vi "Configure CAN Trigger.vi"(0 "VISA resource name":refnum<visa-resource-name>, 1 "Trigger Condition (0: Start of Frame (SOF))":i32(ring) items=["Start of Frame (SOF)", "Data", "Error", "ID Data", "ID Remote", "All Errors", "Overload", "ACK Error", "Message", "MSignal"], 5 "CAN Channel (1: Channel 1)":i32(ring)=1 items=["Channel 1"=1, "Channel 2"=2, "Channel 3"=3, "Channel 4"=4], 7 "Identifier Type (0: Standard)":i32(ring) items=["Standard", "Extended"], 9 "Data Pattern Resource":string="XXXXXXXXXXXXXXXXXXXXXXXXXXXXXXXXXXXXXXXXXXXXXXXXXXXXXXXXXXXXXXXX", 11 "error in (no error)":errorcluster, 12 "Data Pattern Length (8)":i32=8, 13 "Data Pattern ID (XXXXXXXXXXX)":string="XXXXXXXXXXX") -> (4 "VISA resource name out":refnum<visa-resource-name>, 15 "error out":errorcluster)   [LabVIEW 2013, in "Agilent 90000 Series.lvlib"]
doc: "Configures triger values for serial bus.\n\n<b>Notes:</b>\n1. You must set the proper :SBUS<N>:MODE, :SBUS<N>:CAN:TRIGger, and :SBUS<N>:CAN:TRIGger:PATTern:ID:MODE before setting any other trigger values. \n2. This VI is new in firmware version 4.60."
uses:
  Agilent 90000 Series.lvlib
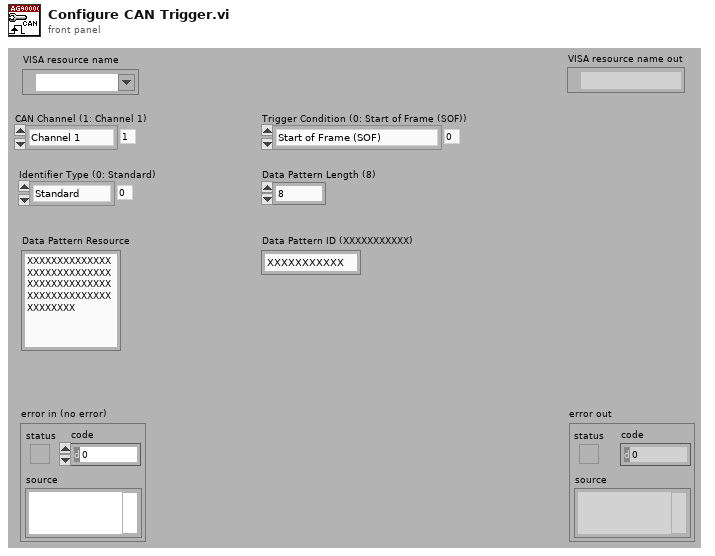
[diagram p1: front panel]
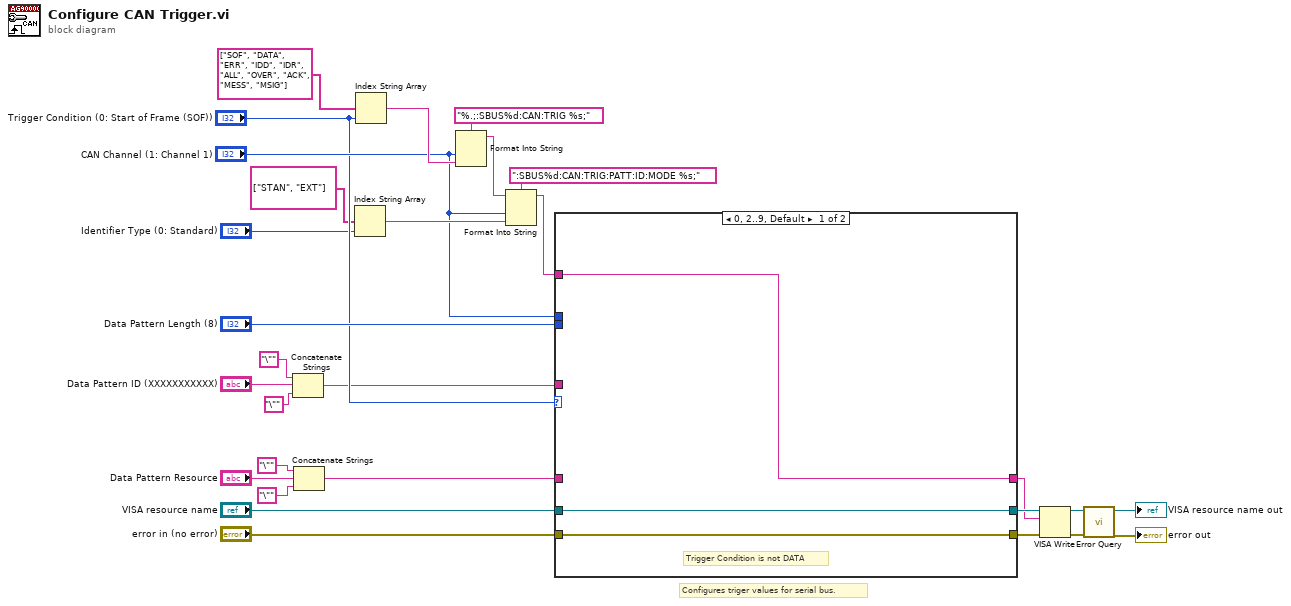
[diagram p0: block diagram]
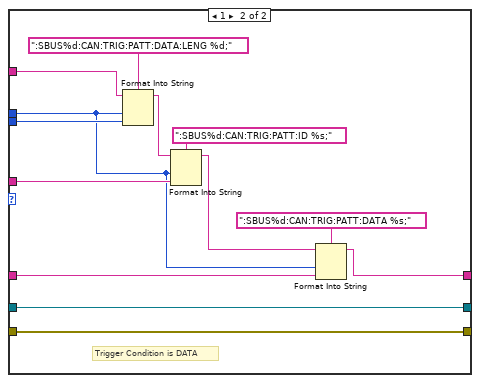
[diagram p2: hidden frame]
diagram:
  # "Configures triger values for serial bus."
  n1 = Concatenate Strings("\"" ("string"), "Data Pattern ID (XXXXXXXXXXX)", "\"" ("string")) -> (w4:string)
  n2 = Concatenate Strings("\"" ("string"), "Data Pattern Resource", "\"" ("string")) -> (w8:string)
  n3 = Index String Array(1:"Identifier Type (0: Standard)", 2:string[] ["STAN", "EXT"] ("string array")) -> (0:w20:string)  [unwired: 1 in]
  n4 = Index String Array(1:"Trigger Condition (0: Start of Frame (SOF))", 2:string[] ["SOF", "DATA", "ERR", "IDD", "IDR", "ALL", "OVER", "ACK", "MESS", "MSIG"] ("string array")) -> (0:w22:string)  [unwired: 1 in]
  n5 = Format Into String(format string="%.;:SBUS%d:CAN:TRIG %s;", "CAN Channel (1: Channel 1)", w22) -> (resulting string=w28:string)  [unwired: 2 in, 1 out]
  n6 = Format Into String(format string=":SBUS%d:CAN:TRIG:PATT:ID:MODE %s;", initial string=w28, "CAN Channel (1: Channel 1)", w20) -> (resulting string=w19:string)  [unwired: 1 in, 1 out]
  n7 = case shown="0, 2..9, Default" "Trigger Condition (0: Start of Frame (SOF))" {
    tunnel: w19 -> [w32 w38]
    tunnel: [w32 w33] -> w10
    tunnel: "Data Pattern Length (8)" -> [_ w42]
    tunnel: "CAN Channel (1: Channel 1)" -> [_ w39]
    tunnel: w4 -> [_ w41]
    tunnel: w8 -> [_ w40]
    tunnel: "VISA resource name" -> [w31 w36]
    tunnel: [w31 w36] -> w15
    tunnel: "error in (no error)" -> [w30 w35]
    tunnel: [w30 w35] -> w13
    frame 0, 2..9, Default {
      # "Trigger Condition is not DATA"
    }
    frame 1 {
      # "Trigger Condition is DATA"
      n8 = Format Into String(format string=":SBUS%d:CAN:TRIG:PATT:DATA:LENG %d;", initial string=w38, w39, w42) -> (resulting string=w45:string)  [unwired: 1 in, 1 out]
      n9 = Format Into String(format string=":SBUS%d:CAN:TRIG:PATT:ID %s;", initial string=w45, w39, w41) -> (resulting string=w43:string)  [unwired: 1 in, 1 out]
      n10 = Format Into String(format string=":SBUS%d:CAN:TRIG:PATT:DATA %s;", initial string=w43, w39, w40) -> (resulting string=w33:string)  [unwired: 1 in, 1 out]
    }
  }
  n11 = VISA Write(VISA resource name=w15, write buffer=w10, error in (no error)=w13) -> (VISA resource name out=w26:refnum<visa-resource-name>, error out=w25:errorcluster)  [unwired: 1 out]
  n12 = call "Error Query.vi"("error in (no error)"=w25, "VISA resource name"=w26) -> ("error out"=→"error out":errorcluster, "VISA resource name out"=→"VISA resource name out":refnum<visa-resource-name>)  [unwired: 6 in, 2 out]
